vi "From Path Cluster.vi"(0 "Pair":cluster{"Key":string, "Value":path}) -> (2 "Map":refnum<class "Map.lvclass">)   [LabVIEW 2018, in "Toolkit.lvlib" / "Data.lvlib" / "Map.lvclass"]
uses:
  Map.lvclass
  Map.lvclass/Map.ctl
  Path/Path.lvclass
  D:/Users/cfield/Code/Field R&D Services/Mustache/LabVIEW/trunk/src/Toolkit/Data/Datum/Datum.lvclass
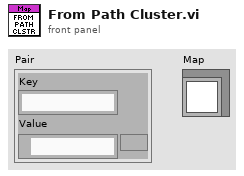
[diagram p1: front panel]
types:
  T1 = cluster{"Key":string, "Path":refnum<class "Path.lvclass">}
  T2 = cluster{"Key":string, "Path":refnum<class "Path.lvclass">}[]
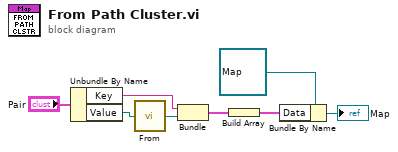
[diagram p0: block diagram]
diagram:
  n1 = Unbundle By Name("Pair") -> ("Key"=w4:string, "Value"=w1:path)
  n2 = call "From.vi"("Value"=w1) -> ("Path"=w3:refnum<class "Path.lvclass">)
  n3 = Bundle("Key"=w4, "Path"=w3) -> (w2:T1)  [unwired: 1 in]
  n4 = Build Array(w2) -> (w6:T2)
  n5 = Bundle By Name(cluster=refnum<class "Map.lvclass"> refnum ("Toolkit.lvlib:Data.lvlib:Map.lvclass"), "Data"=w6) -> (→"Map":refnum<class "Map.lvclass">)
